vi "default value test.vi"() -> ()   [LabVIEW 2013, in "tag bus tests.lvlib"]
uses:
  tag bus tests.lvlib
  tag/Data Type.ctl
  tag/tag descriptor.lvclass/tag descriptor.ctl
  tag/read raw default value.vi
  tag/default value polymorphs/read default value Double.vi
  tag/default value polymorphs/write default value Double.vi
  tag/default value polymorphs/read default value Array of Double.vi
  tag/default value polymorphs/write default value Array of Double.vi
  tag/tag descriptor.lvclass
panel:
  out "dbl[] default read ok":bool
  out "dbl[] default write ok":bool
  out "dbl default write ok":bool
  out "dbl default read ok":bool
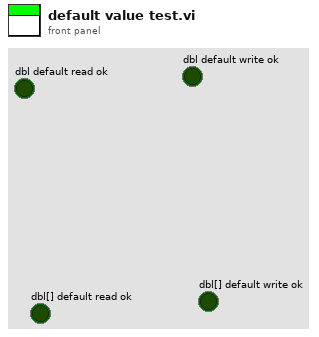
[diagram p1: front panel]
types:
  T1 = typedef "tag bus.lvlib/tag descriptor.lvclass/Data Type.ctl" = enum16{"Double", "Single", "I64", "I32", "I16", "I8", "U64", "U32", "U16", "U8", "Boolean", "String", "Array of Double", "Array of Single", "Array of I64", "Array of I32", "Array of I16", "Array of I8", "Array of U64", "Array of U32", "Array of U16", "Array of U8", "Array of Boolean", "Array of String"}
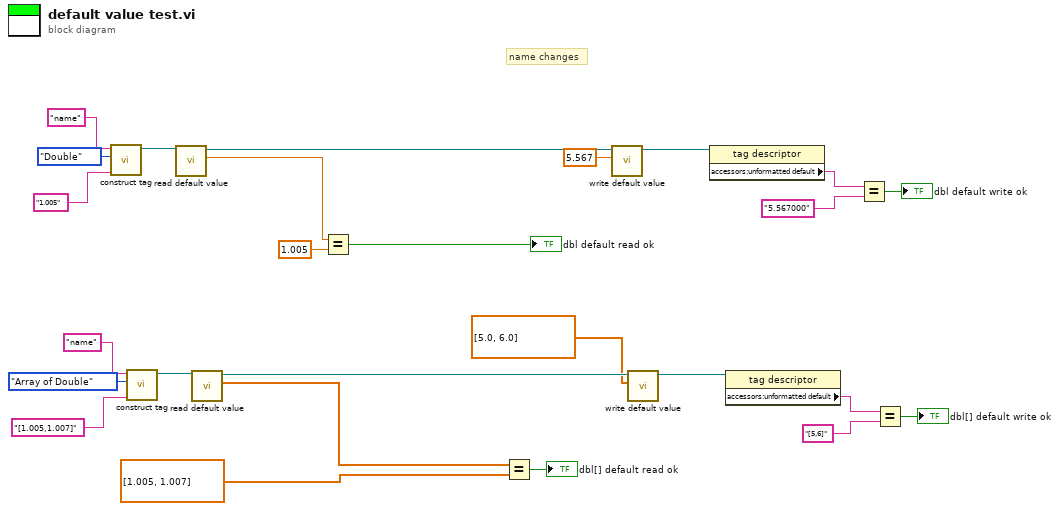
[diagram p0: block diagram]
diagram:
  # "name changes"
  n1 = call "construct tag.vi"("raw default"="1.005", "data type"=Data_Type."Double", "name"="name") -> ("system tag out"=w2:refnum<class "tag descriptor.lvclass">)  [unwired: 8 in]
  n2 = call "construct tag.vi"("raw default"="[1.005,1.007]", "data type"=Data_Type."Array of Double", "name"="name") -> ("system tag out"=w1:refnum<class "tag descriptor.lvclass">)  [unwired: 8 in]
  n3 = call-poly "read default value.vi"("system tag in"=w2) -> ("default value"=w24:dbl, "system tag out"=w21:refnum<class "tag descriptor.lvclass">)  [unwired: 7 in, 2 out]
  n4 = call-poly "read default value.vi"("system tag in"=w1) -> ("default value"=w7:dbl[], "system tag out"=w9:refnum<class "tag descriptor.lvclass">)  [unwired: 7 in, 2 out]
  n5 = Equal?(x=w24, y=1.005) -> (x = y?=→"dbl default read ok":bool)
  n6 = Equal?(x=w7, y=dbl[] [1.005, 1.007]) -> (x = y?=→"dbl[] default read ok":bool)
  n7 = call-poly "write default value.vi"("default value"=5.567, "system tag in"=w21) -> ("system tag out"=w19:refnum<class "tag descriptor.lvclass">)  [unwired: 8 in, 1 out]
  n8 = call-poly "write default value.vi"("default value"=dbl[] [5.0, 6.0], "system tag in"=w9) -> ("system tag out"=w10:refnum<class "tag descriptor.lvclass">)  [unwired: 8 in, 1 out]
  n9 = property class="tag descriptor"(reference=w19) -> ("accessors:unformatted default"=w17:string)  [unwired: 1 in, 2 out]
  n10 = property class="tag descriptor"(reference=w10) -> ("accessors:unformatted default"=w12:string)  [unwired: 1 in, 2 out]
  n11 = Equal?(x=w17, y="5.567000") -> (x = y?=→"dbl default write ok":bool)
  n12 = Equal?(x=w12, y="[5,6]") -> (x = y?=→"dbl[] default write ok":bool)
